vi "Create Member if Invalid Ref.vi"(5 "Additional Scripting Ref":T2, 6 "Scaffold Project Refs":T1, 7 "Member Template":refnum<vi>, 8 "Dynamic?":bool, 9 "Member Name":string, 10 "Parent":refnum<vi>, 11 "Member In":refnum<vi>) -> (3 "Member ProjectItem":refnum<vi>)   [LabVIEW 2018, in "LVClassByRef.lvlib"]
uses:
  <resource>/Framework/Providers/LVClassByRef/LVClassByRef.lvlib
  <resource>/Framework/Providers/LVClassByRef/Additional Scripting Ref.ctl
  <resource>/Framework/Providers/LVClassByRef/Scaffold Project Refs.ctl
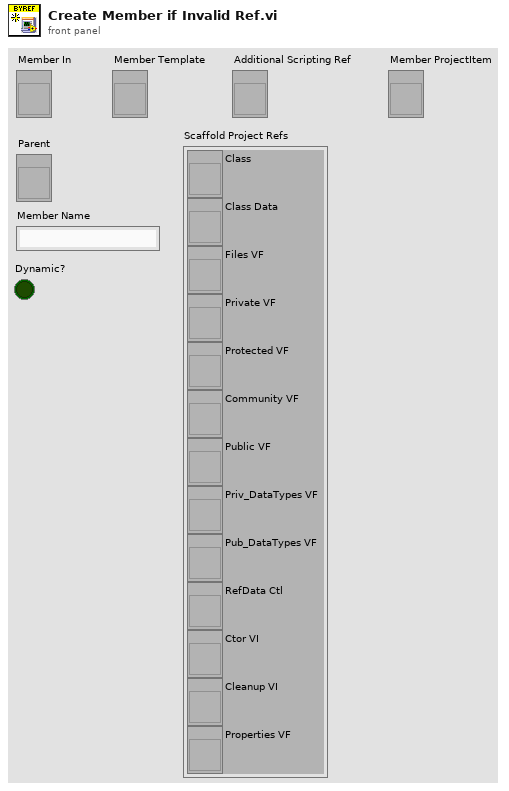
[diagram p1: front panel]
types:
  T1 = typedef "LVClassByRef.lvlib/Scaffold Project Refs.ctl" = cluster{"Class":refnum<vi>, "Class Data":refnum<vi>, "Files VF":refnum<vi>, "Private VF":refnum<vi>, "Protected VF":refnum<vi>, "Community VF":refnum<vi>, "Public VF":refnum<vi>, "Priv_DataTypes VF":refnum<vi>, "Pub_DataTypes VF":refnum<vi>, "RefData Ctl":refnum<vi>, "Ctor VI":refnum<vi>, "Cleanup VI":refnum<vi>, "Properties VF":refnum<vi>}
  T2 = typedef "LVClassByRef.lvlib/Additional Scripting Ref.ctl" = refnum<vi>
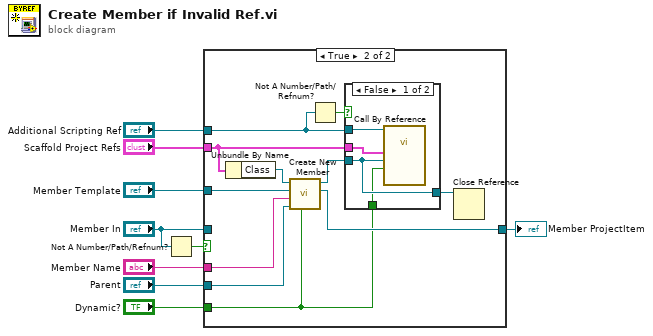
[diagram p0: block diagram]
diagram:
  n1 = Not A Number/Path/Refnum?(number/path/refnum="Member In") -> (NaN/Path/Refnum?=w8:bool)
  n2 = case shown="True" w8 {
    tunnel: "Member In" -> [w10 _]
    tunnel: [w10 w13] -> w7
    tunnel: "Member Template" -> [_ w18]
    tunnel: "Parent" -> [_ w15]
    tunnel: "Member Name" -> [_ w16]
    tunnel: "Additional Scripting Ref" -> [_ w12]
    tunnel: "Scaffold Project Refs" -> [_ w19]
    tunnel: "Dynamic?" -> [_ w11]
    frame False {
    }
    frame True {
      n3 = Unbundle By Name(w19) -> ("Class"=w17:refnum<vi>)
      n4 = call <resource>:"Create New Member.vi"("Dynamic?"=w11, "Parent"=w15, "Name"=w16, "Template"=w18, "LVClassLibrary"=w17) -> ("Member Item"=w13:refnum<vi>, "Member VI"=w14:refnum<vi>)  [unwired: 5 in]
      n5 = Not A Number/Path/Refnum?(number/path/refnum=w12) -> (NaN/Path/Refnum?=w21:bool)
      n6 = case shown="False" w21 {
        tunnel: w14 -> [w23 w26]
        tunnel: w12 -> [w25 _]
        tunnel: [w23 w26] -> w20
        tunnel: w19 -> [w24 _]
        tunnel: w11 -> [w22 _]
        frame False {
          n7 = call-by-ref "?"(reference=w25, "Dynamic"=w22, "VI Refnum"=w23, "Scaffold Project Refs In"=w24) -> ()  [unwired: 9 in, 3 out]
        }
        frame True {
        }
      }
      n8 = Close Reference(reference=w20) -> ()  [unwired: 1 in, 1 out]
    }
  }
  "Member ProjectItem" <- w7
